vi "GetBlockDiagram.vi"() -> (2 "Block Diagram Out":refnum<vi>, 3 "VI Reference Out":refnum<vi>)   [LabVIEW 2012]
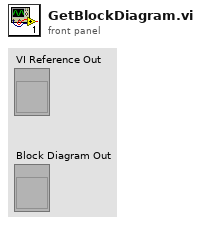
[diagram p1: front panel]
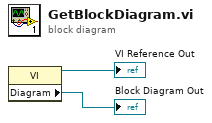
[diagram p0: block diagram]
diagram:
  n1 = property class="VI"() -> (reference out=→"VI Reference Out":refnum<vi>, "Diagram"=→"Block Diagram Out":refnum<vi>)  [unwired: 2 in, 1 out]
